vi "AutoRun.vi"() -> ()   [LabVIEW 2012]
uses:
  resultShow.vi
panel:
  in  "布尔":bool
  out "毫秒计时值":u32
  in  "stepMotor/ECU":string
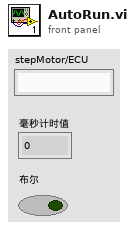
[diagram p1: front panel]
types:
  T1 = cluster{"takesTime":refnum<vi>, "userStatus":refnum<vi>, "userName":refnum<vi>, "connectionMode":refnum<vi>, "productsName":refnum<vi>, "rigStatus":refnum<vi>, "总成扫码":refnum<vi>}
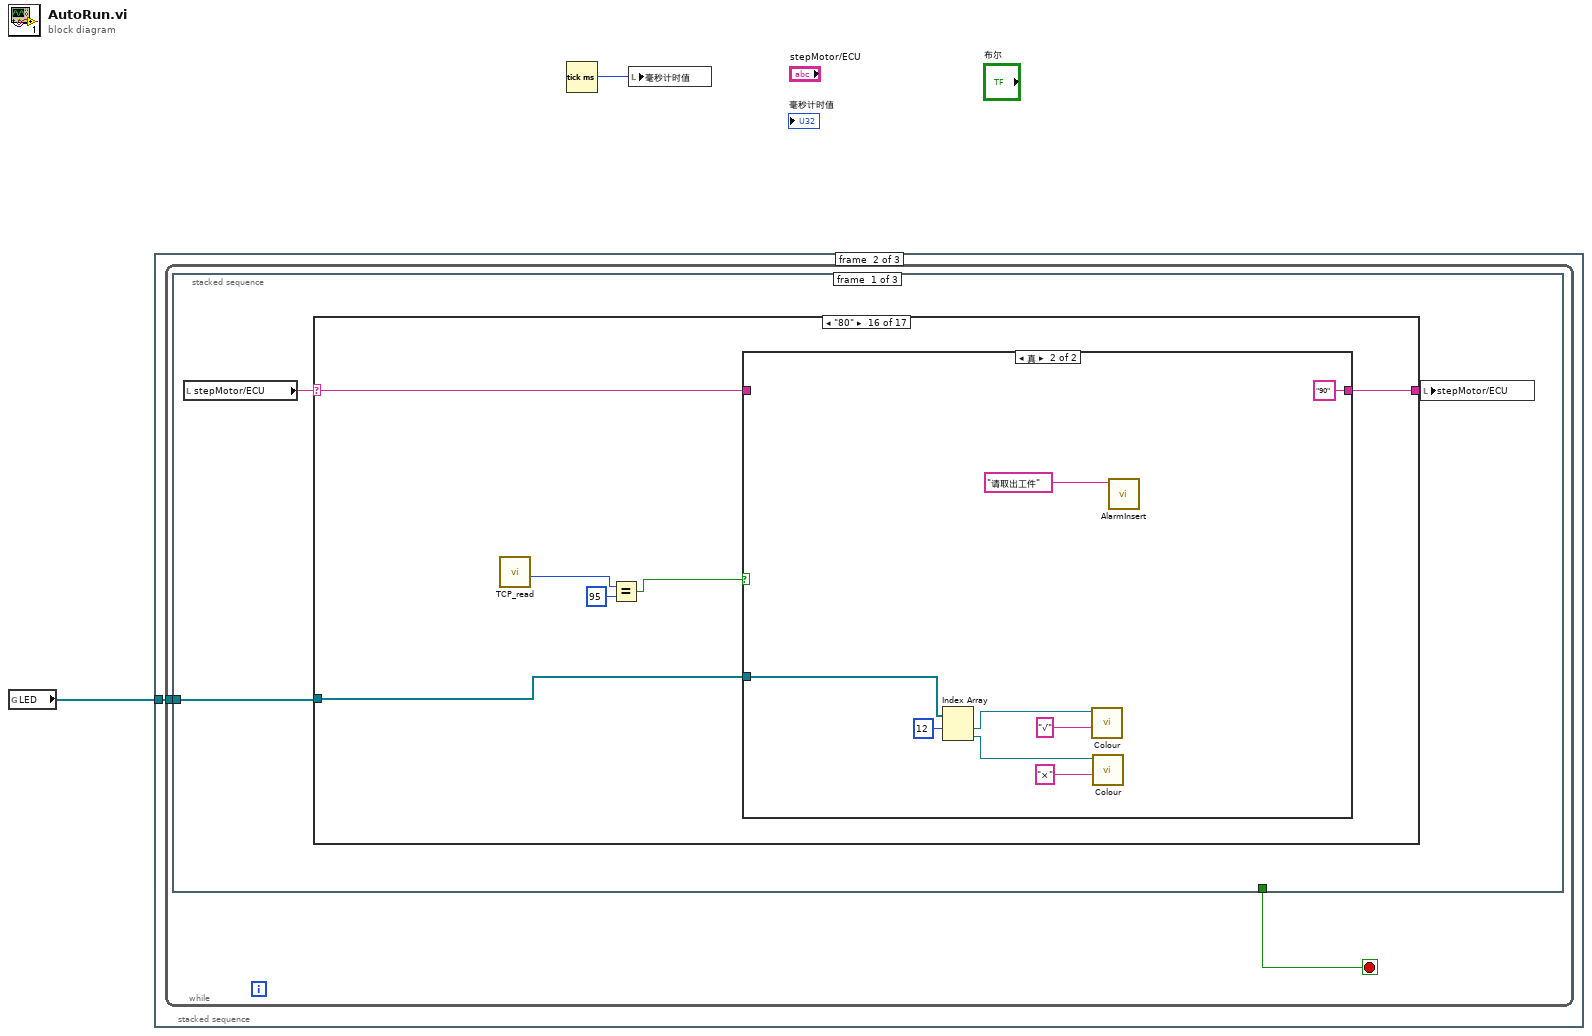
[diagram p0: block diagram]
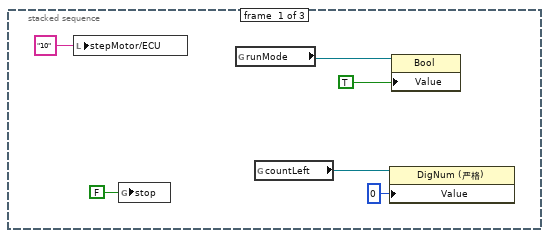
[diagram p2: hidden frame]
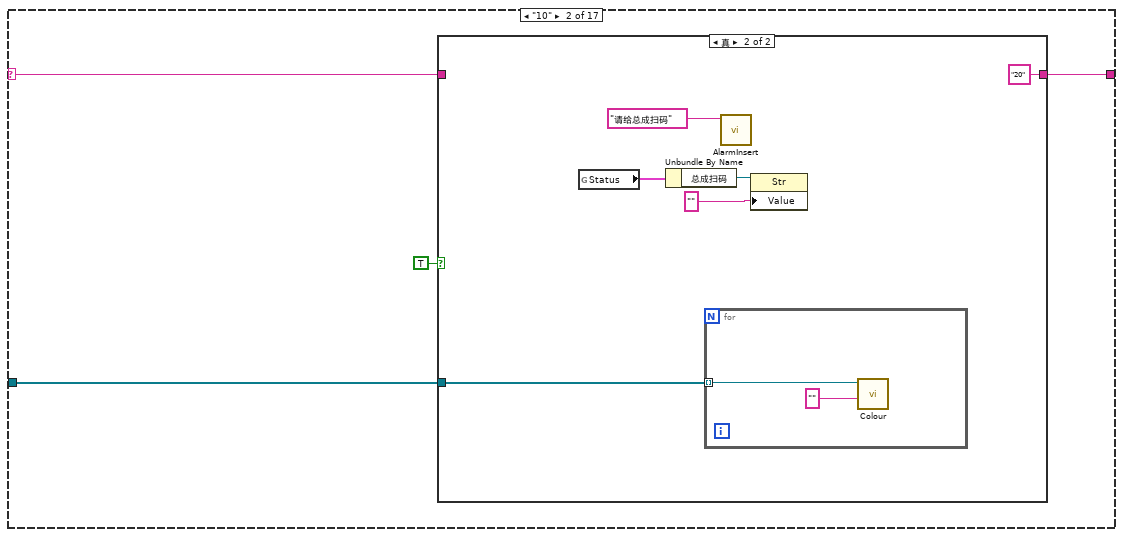
[diagram p4: hidden frame]
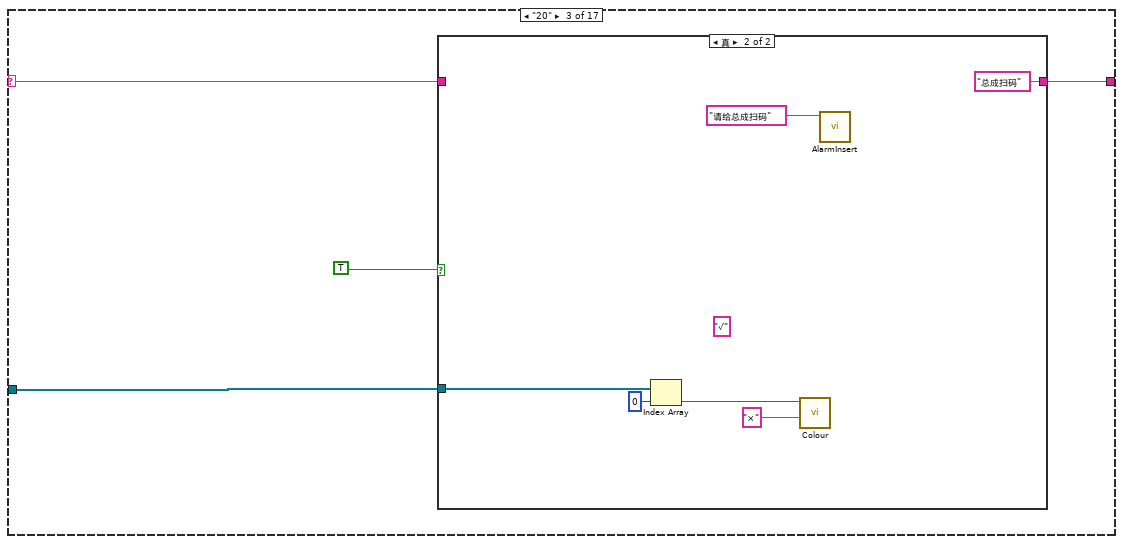
[diagram p6: hidden frame]
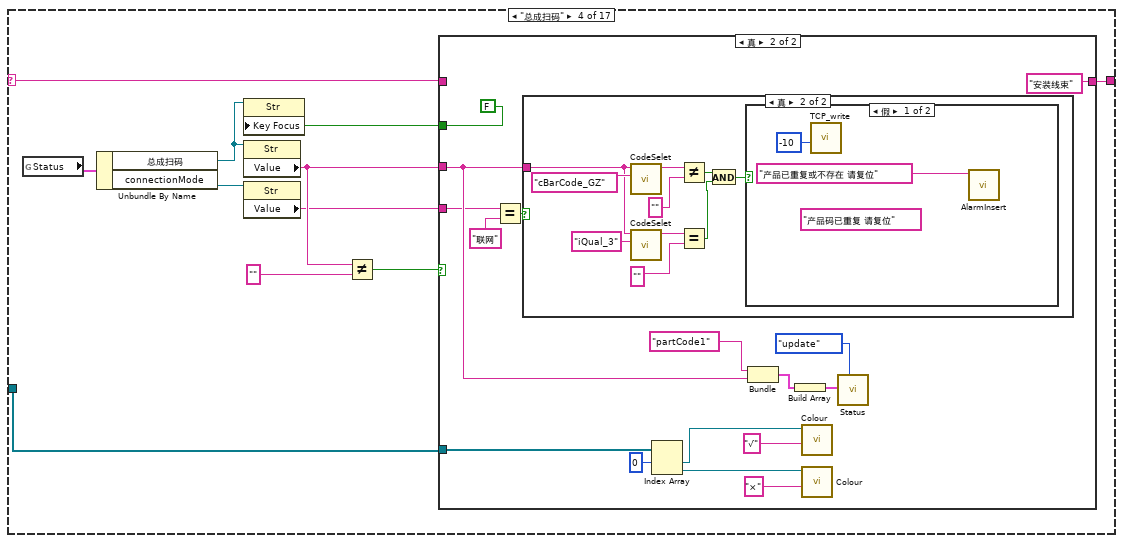
[diagram p8: hidden frame]
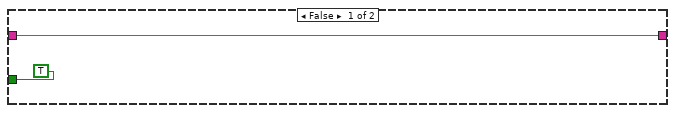
[diagram p9: hidden frame]
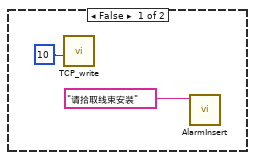
[diagram p10: hidden frame]
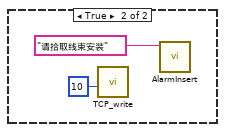
[diagram p11: hidden frame]
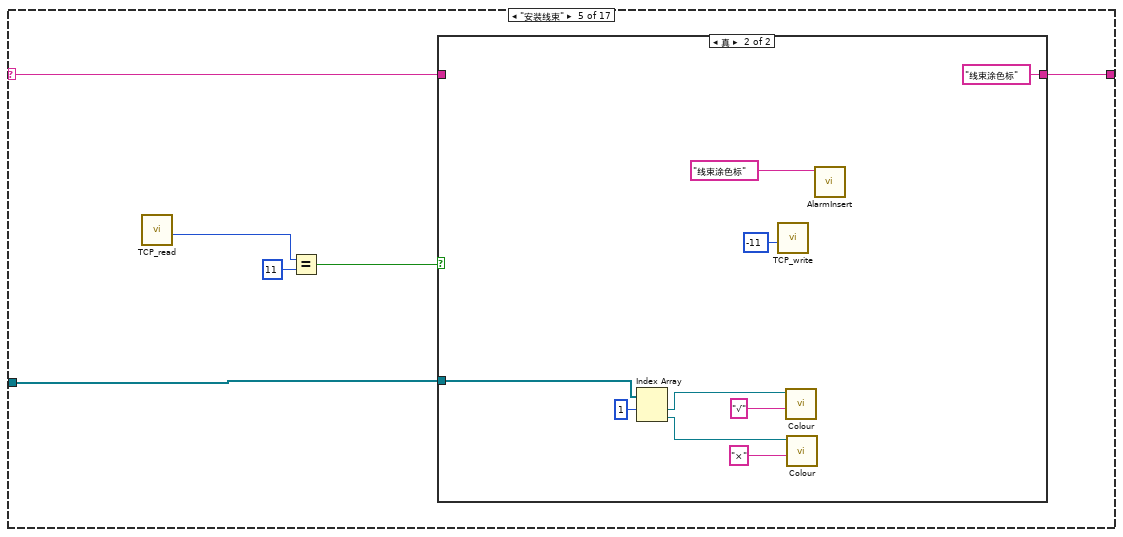
[diagram p12: hidden frame]
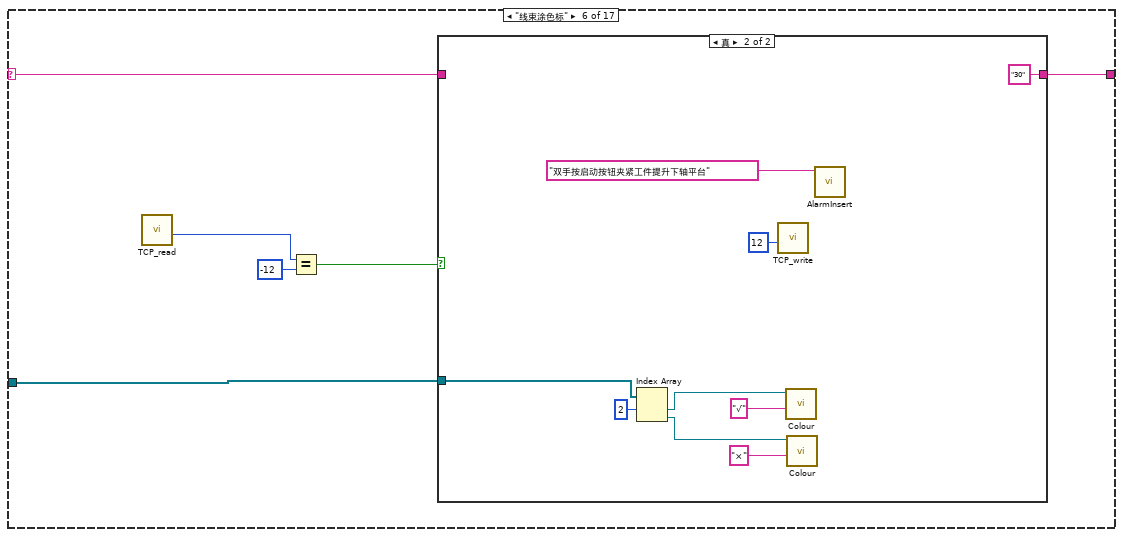
[diagram p14: hidden frame]
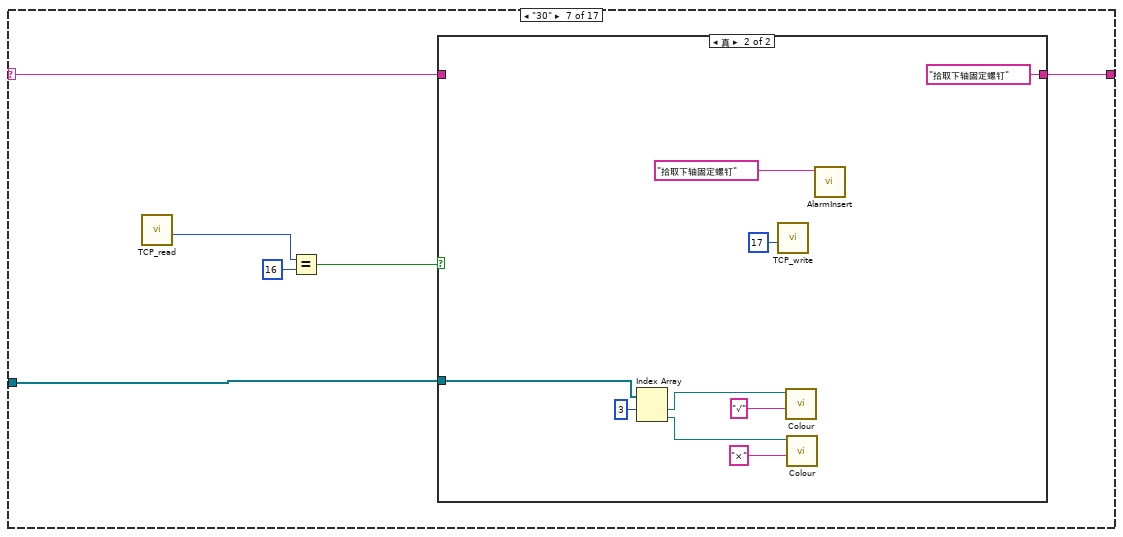
[diagram p16: hidden frame]
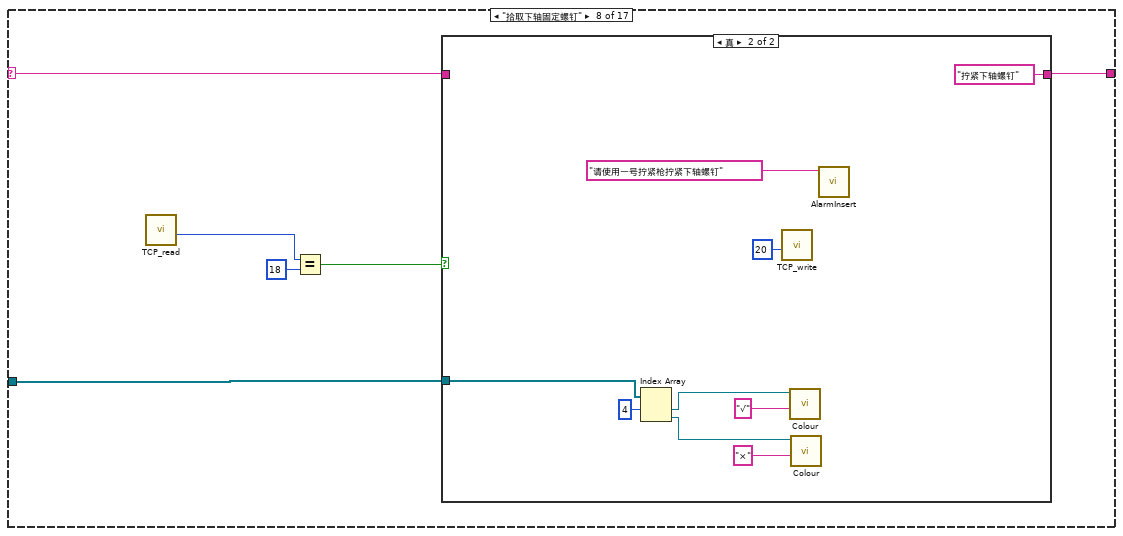
[diagram p18: hidden frame]
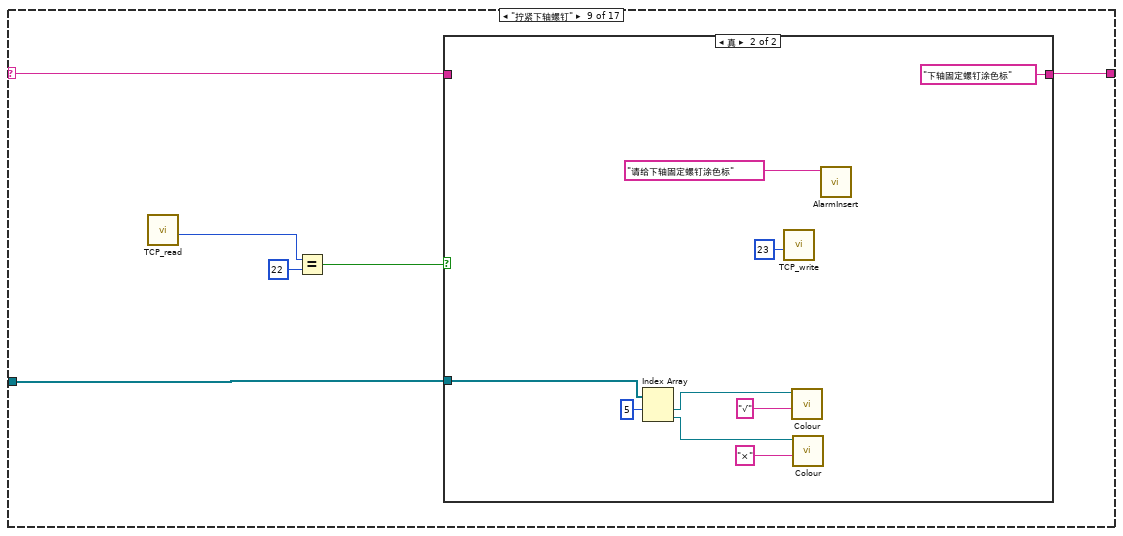
[diagram p20: hidden frame]
diagram:
  n1 = global read "resultShow.vi" "LED"() -> (w2:refnum<vi>[])
  n2 = stacked-sequence {
    tunnel: w2 -> [_ w9 _]
    frame #0 {
      n3 = local write "stepMotor/ECU"("10" ("step")) -> ()
      n4 = global write "全局 3.vi" "stop"(FALSE ("布尔 2")) -> ()
      n5 = global read "resultShow.vi" "runMode"() -> (w5:refnum<vi>)
      n6 = global read "resultShow.vi" "countLeft"() -> (w3:refnum<vi>)
      n7 = property class="DigNum (严格)"(reference=w3, "Value"=u32 0 ("值")) -> ()  [unwired: 1 in, 2 out]
      n8 = property class="Bool"(reference=w5, "Value"=TRUE ("m")) -> ()  [unwired: 1 in, 2 out]
    }
    frame #1 {
      n9 = while {
        tunnel: w9 -> [w10]
        stop <- w11 stop-if-true
        n10 = stacked-sequence {
          tunnel: [_ _ w333] -> w11
          tunnel: w10 -> [w12 _ _]
          frame #0 {
            n11 = local read "stepMotor/ECU"() -> (w13:string)
            n12 = case shown="\"80\"" w13 {
              selector: w13 -> [w15 w18 w31 w46 w89 w105 w121 w134 w150 w167 w185 w201 w217 w231 w247 w274 w289]
              tunnel: [w15 w19 w32 w44 w90 w106 w122 w133 w151 w165 w186 w202 w218 w229 w248 w275 w290] -> w14
              tunnel: w12 -> [_ w16 w30 w45 w85 w101 w117 w135 w149 w166 w181 w197 w213 w230 w246 w270 w285]
              frame "假", Default {
              }
              frame "10" {
                n13 = case shown="真" TRUE {
                  tunnel: [w20 "20"] -> w19
                  tunnel: w18 -> [w20 _]
                  tunnel: w16 -> [_ w25]
                  frame False {
                  }
                  frame True {
                    n14 = global read "resultShow.vi" "Status"() -> (w22:T1)
                    n15 = Unbundle By Name(w22) -> ("总成扫码"=w23:refnum<vi>)
                    n16 = for {
                      tunnel: w25 -> [w27] mode=indexing
                      n17 = call "Colour.vi"("result"="" ("元素"), "colourRef"=w27) -> ()  [unwired: 9 in, 1 out]
                    }
                    n18 = call "AlarmInsert.vi"("消息名"="请给总成扫码") -> ()  [unwired: 11 in]
                    n19 = property class="Str"(reference=w23, "Value"="") -> ()  [unwired: 1 in, 2 out]
                  }
                }
              }
              frame "20" {
                n20 = case shown="真" TRUE {
                  tunnel: [w33 "总成扫码"] -> w32
                  tunnel: w31 -> [w33 _]
                  tunnel: w30 -> [_ w35]
                  frame False {
                  }
                  frame True {
                    (unwired) "√" ("元素")
                    n21 = Index Array(array=w35, index=0 ("索引")) -> (element=w37:refnum<vi>)
                    n22 = call "Colour.vi"("result"="×" ("元素"), "colourRef"=w37) -> ()  [unwired: 9 in, 1 out]
                    n23 = call "AlarmInsert.vi"("消息名"="请给总成扫码") -> ()  [unwired: 11 in]
                  }
                }
              }
              frame "总成扫码" {
                n24 = global read "resultShow.vi" "Status"() -> (w47:T1)
                n25 = Unbundle By Name(w47) -> ("总成扫码"=w49:refnum<vi>, "connectionMode"=w41:refnum<vi>)
                n26 = property class="Str"(reference=w49) -> ("Value"=w43:string)  [unwired: 1 in, 2 out]
                n27 = property class="Str"(reference=w41) -> ("Value"=w40:string)  [unwired: 1 in, 2 out]
                n28 = Not Equal?(x=w43, y="") -> (x != y?=w50:bool)
                n29 = case shown="真" w50 {
                  tunnel: [w52 "安装线束"] -> w44
                  tunnel: w46 -> [w52 _]
                  tunnel: w45 -> [_ w65]
                  tunnel: w43 -> [_ w59]
                  tunnel: [TRUE FALSE] -> w42
                  tunnel: w40 -> [_ w53]
                  frame False {
                  }
                  frame True {
                    n30 = Equal?(x=w53, y="联网") -> (x = y?=w55:bool)
                    n31 = case shown="真" w55 {
                      tunnel: w59 -> [_ w76]
                      frame False {
                        n32 = call "TCP_write.vi"("写入数据"=i8 10) -> ()  [unwired: 11 in]
                        n33 = call "AlarmInsert.vi"("消息名"="请拾取线束安装") -> ()  [unwired: 11 in]
                      }
                      frame True {
                        n34 = call "CodeSelet.vi"("字符串"="cBarCode_GZ" ("code"), "parameter name"=w76) -> ("readData"=w79:string)  [unwired: 9 in]
                        n35 = call "CodeSelet.vi"("字符串"="iQual_3" ("code"), "parameter name"=w76) -> ("readData"=w77:string)  [unwired: 9 in]
                        n36 = Not Equal?(x=w79, y="" ("元素")) -> (x != y?=w74:bool)
                        n37 = Equal?(x=w77, y="" ("元素")) -> (x = y?=w72:bool)
                        n38 = And(x=w74, y=w72) -> (x .and. y?=w73:bool)
                        n39 = case shown="假" w73 {
                          frame False {
                            (unwired) "产品码已重复 请复位" ("string_5")
                            n40 = call "TCP_write.vi"("写入数据"=i8 -10) -> ()  [unwired: 11 in]
                            n41 = call "AlarmInsert.vi"("消息名"="产品已重复或不存在 请复位" ("string_5")) -> ()  [unwired: 11 in]
                          }
                          frame True {
                            n42 = call "TCP_write.vi"("写入数据"=i8 10) -> ()  [unwired: 11 in]
                            n43 = call "AlarmInsert.vi"("消息名"="请拾取线束安装") -> ()  [unwired: 11 in]
                          }
                        }
                      }
                    }
                    n44 = Index Array(array=w65, index #1=0 ("索引")) -> (element #1=w63:refnum<vi>, element #2=w62:refnum<vi>)  [unwired: 1 in]
                    n45 = Bundle("元素"="partCode1", "Value"=w59) -> (w61:cluster{"元素":string, "Value":string})  [unwired: 1 in]
                    n46 = Build Array(w61) -> (w58:cluster{"元素":string, "Value":string}[])
                    n47 = call "Colour.vi"("result"="√" ("元素"), "colourRef"=w63) -> ()  [unwired: 9 in, 1 out]
                    n48 = call "Colour.vi"("result"="×" ("元素"), "colourRef"=w62) -> ()  [unwired: 9 in, 1 out]
                    n49 = call "Status.vi"("模式"=enum16{"select", "insert", "update", "delete"}."update", "nameData"=w58) -> ()  [unwired: 9 in, 1 out]
                  }
                }
                n50 = property class="Str"(reference=w49, "Key Focus"=w42) -> ()  [unwired: 1 in, 2 out]
              }
              frame "安装线束" {
                n51 = call "TCP_read.vi"() -> ("元素"=w88:i8)  [unwired: 10 in, 1 out]
                n52 = Equal?(x=w88, y=i8 11) -> (x = y?=w86:bool)
                n53 = case shown="真" w86 {
                  tunnel: [w91 "线束涂色标"] -> w90
                  tunnel: w89 -> [w91 _]
                  tunnel: w85 -> [_ w92]
                  frame False {
                  }
                  frame True {
                    n54 = Index Array(array=w92, index #1=1 ("索引")) -> (element #1=w96:refnum<vi>, element #2=w93:refnum<vi>)  [unwired: 1 in]
                    n55 = call "TCP_write.vi"("写入数据"=i8 -11) -> ()  [unwired: 11 in]
                    n56 = call "Colour.vi"("result"="√" ("元素"), "colourRef"=w96) -> ()  [unwired: 9 in, 1 out]
                    n57 = call "Colour.vi"("result"="×" ("元素"), "colourRef"=w93) -> ()  [unwired: 9 in, 1 out]
                    n58 = call "AlarmInsert.vi"("消息名"="线束涂色标" ("string_5")) -> ()  [unwired: 11 in]
                  }
                }
              }
              frame "线束涂色标" {
                n59 = call "TCP_read.vi"() -> ("元素"=w104:i8)  [unwired: 10 in, 1 out]
                n60 = Equal?(x=w104, y=i8 -12) -> (x = y?=w102:bool)
                n61 = case shown="真" w102 {
                  tunnel: [w107 "30"] -> w106
                  tunnel: w105 -> [w107 _]
                  tunnel: w101 -> [_ w108]
                  frame False {
                  }
                  frame True {
                    n62 = Index Array(array=w108, index #1=2 ("索引")) -> (element #1=w112:refnum<vi>, element #2=w109:refnum<vi>)  [unwired: 1 in]
                    n63 = call "TCP_write.vi"("写入数据"=i8 12) -> ()  [unwired: 11 in]
                    n64 = call "Colour.vi"("result"="√" ("元素"), "colourRef"=w112) -> ()  [unwired: 9 in, 1 out]
                    n65 = call "Colour.vi"("result"="×" ("元素"), "colourRef"=w109) -> ()  [unwired: 9 in, 1 out]
                    n66 = call "AlarmInsert.vi"("消息名"="双手按启动按钮夹紧工件提升下轴平台" ("string_5")) -> ()  [unwired: 11 in]
                  }
                }
              }
              frame "30" {
                n67 = call "TCP_read.vi"() -> ("元素"=w120:i8)  [unwired: 10 in, 1 out]
                n68 = Equal?(x=w120, y=i8 16) -> (x = y?=w118:bool)
                n69 = case shown="真" w118 {
                  tunnel: [w123 "拾取下轴固定螺钉"] -> w122
                  tunnel: w121 -> [w123 _]
                  tunnel: w117 -> [_ w124]
                  frame False {
                  }
                  frame True {
                    n70 = Index Array(array=w124, index #1=3 ("索引")) -> (element #1=w128:refnum<vi>, element #2=w125:refnum<vi>)  [unwired: 1 in]
                    n71 = call "TCP_write.vi"("写入数据"=i8 17) -> ()  [unwired: 11 in]
                    n72 = call "Colour.vi"("result"="√" ("元素"), "colourRef"=w128) -> ()  [unwired: 9 in, 1 out]
                    n73 = call "Colour.vi"("result"="×" ("元素"), "colourRef"=w125) -> ()  [unwired: 9 in, 1 out]
                    n74 = call "AlarmInsert.vi"("消息名"="拾取下轴固定螺钉" ("string_5")) -> ()  [unwired: 11 in]
                  }
                }
              }
              frame "拾取下轴固定螺钉" {
                n75 = call "TCP_read.vi"() -> ("元素"=w136:i8)  [unwired: 10 in, 1 out]
                n76 = Equal?(x=w136, y=i8 18) -> (x = y?=w138:bool)
                n77 = case shown="真" w138 {
                  tunnel: [w139 "拧紧下轴螺钉"] -> w133
                  tunnel: w134 -> [w139 _]
                  tunnel: w135 -> [_ w140]
                  frame False {
                  }
                  frame True {
                    n78 = Index Array(array=w140, index #1=4 ("索引")) -> (element #1=w144:refnum<vi>, element #2=w141:refnum<vi>)  [unwired: 1 in]
                    n79 = call "TCP_write.vi"("写入数据"=i8 20) -> ()  [unwired: 11 in]
                    n80 = call "Colour.vi"("result"="√" ("元素"), "colourRef"=w144) -> ()  [unwired: 9 in, 1 out]
                    n81 = call "Colour.vi"("result"="×" ("元素"), "colourRef"=w141) -> ()  [unwired: 9 in, 1 out]
                    n82 = call "AlarmInsert.vi"("消息名"="请使用一号拧紧枪拧紧下轴螺钉" ("string_5")) -> ()  [unwired: 11 in]
                  }
                }
              }
              frame "拧紧下轴螺钉" {
                n83 = call "TCP_read.vi"() -> ("元素"=w152:i8)  [unwired: 10 in, 1 out]
                n84 = Equal?(x=w152, y=i8 22) -> (x = y?=w154:bool)
                n85 = case shown="真" w154 {
                  tunnel: [w155 "下轴固定螺钉涂色标"] -> w151
                  tunnel: w150 -> [w155 _]
                  tunnel: w149 -> [_ w156]
                  frame False {
                  }
                  frame True {
                    n86 = Index Array(array=w156, index #1=5 ("索引")) -> (element #1=w160:refnum<vi>, element #2=w157:refnum<vi>)  [unwired: 1 in]
                    n87 = call "TCP_write.vi"("写入数据"=i8 23) -> ()  [unwired: 11 in]
                    n88 = call "Colour.vi"("result"="√" ("元素"), "colourRef"=w160) -> ()  [unwired: 9 in, 1 out]
                    n89 = call "Colour.vi"("result"="×" ("元素"), "colourRef"=w157) -> ()  [unwired: 9 in, 1 out]
                    n90 = call "AlarmInsert.vi"("消息名"="请给下轴固定螺钉涂色标" ("string_5")) -> ()  [unwired: 11 in]
                  }
                }
              }
              frame "下轴固定螺钉涂色标" {
                n91 = call "TCP_read.vi"() -> ("元素"=w168:i8)  [unwired: 10 in, 1 out]
                n92 = Equal?(x=w168, y=i8 24) -> (x = y?=w170:bool)
                n93 = case shown="真" w170 {
                  tunnel: [w171 "40"] -> w165
                  tunnel: w167 -> [w171 _]
                  tunnel: w166 -> [_ w172]
                  frame False {
                  }
                  frame True {
                    n94 = Index Array(array=w172, index #1=6 ("索引")) -> (element #1=w176:refnum<vi>, element #2=w173:refnum<vi>)  [unwired: 1 in]
                    n95 = call "TCP_write.vi"("写入数据"=i8 25) -> ()  [unwired: 11 in]
                    n96 = call "Colour.vi"("result"="√" ("元素"), "colourRef"=w176) -> ()  [unwired: 9 in, 1 out]
                    n97 = call "Colour.vi"("result"="×" ("元素"), "colourRef"=w173) -> ()  [unwired: 9 in, 1 out]
                    n98 = call "AlarmInsert.vi"("消息名"="请将下轴翻起后按左启动键复位下轴平台" ("string_5")) -> ()  [unwired: 11 in]
                  }
                }
              }
              frame "40" {
                n99 = call "TCP_read.vi"() -> ("元素"=w184:i8)  [unwired: 10 in, 1 out]
                n100 = Equal?(x=w184, y=i8 31) -> (x = y?=w182:bool)
                n101 = case shown="真" w182 {
                  tunnel: [w187 "50"] -> w186
                  tunnel: w185 -> [w187 _]
                  tunnel: w181 -> [_ w188]
                  frame False {
                  }
                  frame True {
                    n102 = Index Array(array=w188, index #1=7 ("索引")) -> (element #1=w192:refnum<vi>, element #2=w189:refnum<vi>)  [unwired: 1 in]
                    n103 = call "TCP_write.vi"("写入数据"=i8 40) -> ()  [unwired: 11 in]
                    n104 = call "AlarmInsert.vi"("消息名"="双手按启动按钮启动翻转" ("string_5")) -> ()  [unwired: 11 in]
                    n105 = call "Colour.vi"("result"="√" ("元素"), "colourRef"=w192) -> ()  [unwired: 9 in, 1 out]
                    n106 = call "Colour.vi"("result"="×" ("元素"), "colourRef"=w189) -> ()  [unwired: 9 in, 1 out]
                  }
                }
              }
              frame "50" {
                n107 = call "TCP_read.vi"() -> ("元素"=w200:i8)  [unwired: 10 in, 1 out]
                n108 = Equal?(x=w200, y=i8 43) -> (x = y?=w198:bool)
                n109 = case shown="真" w198 {
                  tunnel: [w203 "60"] -> w202
                  tunnel: w201 -> [w203 _]
                  tunnel: w197 -> [_ w204]
                  frame False {
                  }
                  frame True {
                    n110 = Index Array(array=w204, index #1=8 ("索引")) -> (element #1=w208:refnum<vi>, element #2=w205:refnum<vi>)  [unwired: 1 in]
                    n111 = call "TCP_write.vi"("写入数据"=i8 50) -> ()  [unwired: 11 in]
                    n112 = call "Colour.vi"("result"="√" ("元素"), "colourRef"=w208) -> ()  [unwired: 9 in, 1 out]
                    n113 = call "Colour.vi"("result"="×" ("元素"), "colourRef"=w205) -> ()  [unwired: 9 in, 1 out]
                    n114 = call "AlarmInsert.vi"("消息名"="请向左边转两圈以上" ("string_5")) -> ()  [unwired: 11 in]
                  }
                }
              }
              frame "60" {
                n115 = call "TCP_read.vi"() -> ("元素"=w216:i8)  [unwired: 10 in, 1 out]
                n116 = Equal?(x=w216, y=i8 51) -> (x = y?=w214:bool)
                n117 = case shown="真" w214 {
                  tunnel: [w219 "61"] -> w218
                  tunnel: w217 -> [w219 _]
                  tunnel: w213 -> [_ w220]
                  frame False {
                  }
                  frame True {
                    n118 = Index Array(array=w220, index #1=9 ("索引")) -> (element #1=w224:refnum<vi>, element #2=w221:refnum<vi>)  [unwired: 1 in]
                    n119 = call "TCP_write.vi"("写入数据"=i8 60) -> ()  [unwired: 11 in]
                    n120 = call "Colour.vi"("result"="√" ("元素"), "colourRef"=w224) -> ()  [unwired: 9 in, 1 out]
                    n121 = call "Colour.vi"("result"="×" ("元素"), "colourRef"=w221) -> ()  [unwired: 9 in, 1 out]
                    n122 = call "AlarmInsert.vi"("消息名"="请向右边转两圈以上" ("string_5")) -> ()  [unwired: 11 in]
                  }
                }
              }
              frame "61" {
                n123 = call "TCP_read.vi"() -> ("元素"=w234:i8)  [unwired: 10 in, 1 out]
                n124 = Equal?(x=w234, y=i8 61) -> (x = y?=w232:bool)
                n125 = case shown="真" w232 {
                  tunnel: [w235 "70"] -> w229
                  tunnel: w231 -> [w235 _]
                  tunnel: w230 -> [_ w236]
                  frame False {
                  }
                  frame True {
                    n126 = Index Array(array=w236, index #1=10 ("索引")) -> (element #1=w240:refnum<vi>, element #2=w237:refnum<vi>)  [unwired: 1 in]
                    n127 = call "TCP_write.vi"("写入数据"=i8 62) -> ()  [unwired: 11 in]
                    n128 = call "Colour.vi"("result"="√" ("元素"), "colourRef"=w240) -> ()  [unwired: 9 in, 1 out]
                    n129 = call "Colour.vi"("result"="×" ("元素"), "colourRef"=w237) -> ()  [unwired: 9 in, 1 out]
                    n130 = call "AlarmInsert.vi"("消息名"="请判断是否合格" ("string_5")) -> ()  [unwired: 11 in]
                  }
                }
              }
              frame "70" {
                n131 = call "TCP_read.vi"() -> ("元素"=w245:i8)  [unwired: 10 in, 1 out]
                n132 = case shown="72" w245 {
                  tunnel: [w249 w252 w261 "80"] -> w248
                  tunnel: w247 -> [w249 w252 w261 _]
                  tunnel: w246 -> [_ w253 w262 _]
                  frame Default {
                  }
                  frame 71 {
                    n133 = Index Array(array=w253, index #1=11 ("索引")) -> (element #1=w257:refnum<vi>, element #2=w254:refnum<vi>)  [unwired: 1 in]
                    n134 = global write "全局 3.vi" "总合格状态"("" ("元素")) -> ()
                    n135 = global write "全局 3.vi" "合格判断"("√" ("元素")) -> ()
                    n136 = call "Colour.vi"("result"="√" ("元素"), "colourRef"=w257) -> ()  [unwired: 9 in, 1 out]
                    n137 = call "Colour.vi"("result"="×" ("元素"), "colourRef"=w254) -> ()  [unwired: 9 in, 1 out]
                    n138 = call "AlarmInsert.vi"("消息名"="合格 请拆卸下轴后双手按启动按钮" ("string_5")) -> ()  [unwired: 11 in]
                  }
                  frame 72 {
                    w260 = "×" ("元素")
                    n139 = Index Array(array=w262, index #1=11 ("索引")) -> (element #1=w266:refnum<vi>, element #2=w263:refnum<vi>)  [unwired: 1 in]
                    n140 = global write "全局 3.vi" "总合格状态"(w260) -> ()
                    n141 = global write "全局 3.vi" "合格判断"(w260) -> ()
                    n142 = call "Colour.vi"("result"="×" ("元素"), "colourRef"=w266) -> ()  [unwired: 9 in, 1 out]
                    n143 = call "Colour.vi"("result"="×" ("元素"), "colourRef"=w263) -> ()  [unwired: 9 in, 1 out]
                    n144 = call "AlarmInsert.vi"("消息名"="不合格 请拆卸下轴后双手按启动按钮" ("string_5")) -> ()  [unwired: 11 in]
                  }
                  frame 81 {
                  }
                }
              }
              frame "80" {
                n145 = call "TCP_read.vi"() -> ("元素"=w273:i8)  [unwired: 10 in, 1 out]
                n146 = Equal?(x=w273, y=i8 95) -> (x = y?=w271:bool)
                n147 = case shown="真" w271 {
                  tunnel: [w276 "90"] -> w275
                  tunnel: w274 -> [w276 _]
                  tunnel: w270 -> [_ w278]
                  frame False {
                  }
                  frame True {
                    n148 = Index Array(array=w278, index #1=12 ("索引")) -> (element #1=w282:refnum<vi>, element #2=w279:refnum<vi>)  [unwired: 1 in]
                    n149 = call "Colour.vi"("result"="√" ("元素"), "colourRef"=w282) -> ()  [unwired: 9 in, 1 out]
                    n150 = call "Colour.vi"("result"="×" ("元素"), "colourRef"=w279) -> ()  [unwired: 9 in, 1 out]
                    n151 = call "AlarmInsert.vi"("消息名"="请取出工件" ("string_5")) -> ()  [unwired: 11 in]
                  }
                }
              }
              frame "90" {
                n152 = call "TCP_read.vi"() -> ("元素"=w288:i8)  [unwired: 10 in, 1 out]
                n153 = Equal?(x=w288, y=i8 95) -> (x = y?=w286:bool)
                n154 = case shown="真" w286 {
                  tunnel: [w291 "10"] -> w290
                  tunnel: w289 -> [w291 _]
                  tunnel: w285 -> [_ w310]
                  frame False {
                  }
                  frame True {
                    n155 = global read "resultShow.vi" "Status"() -> (w303:T1)
                    n156 = global read "resultShow.vi" "countLeft"() -> (w309:refnum<vi>)
                    n157 = local read "毫秒计时值"() -> (w294:u32)
                    n158 = Tick Count (ms)() -> (millisecond timer value=w292:u32)
                    n159 = Unbundle By Name(w303) -> ("connectionMode"=w304:refnum<vi>)
                    n160 = Index Array(array=w310, index=13 ("索引")) -> (element=w312:refnum<vi>)
                    n161 = Subtract(x=w292, y=w294) -> (x-y=w298:u32)
                    n162 = property class="DigNum (严格)"(reference=w309) -> (reference out=w308:refnum<vi>, "Value"=w307:u32)  [unwired: 1 in, 1 out]
                    n163 = Divide(x=w298, y=u32 1000) -> (x/y=w296:dbl)
                    n164 = property class="Str"(reference=w304) -> ("Value"=w301:string)  [unwired: 1 in, 2 out]
                    n165 = To Time Stamp(1:w296) -> (0:w295:timestamp)
                    n166 = call "Colour.vi"("result"="√" ("元素"), "colourRef"=w312) -> ()  [unwired: 9 in, 1 out]
                    n167 = Format Date/Time String(seconds (now)=w295) -> (date/time string=w293:string)  [unwired: 2 in]
                    n168 = Increment(x=w307) -> (x+1=w306:u32)
                    n169 = Equal?(x=w301, y="联网") -> (x = y?=w302:bool)
                    n170 = case shown="真" w302 {
                      frame False {
                      }
                      frame True {
                        n171 = call "updateiqual.vi"() -> ()  [unwired: 11 in]
                      }
                    }
                    n172 = property class="DigNum (严格)"(reference=w308, "Value"=w306) -> ()  [unwired: 1 in, 2 out]
                    n173 = call "AlarmInsert.vi"("takesTime"=w293, "消息名"="完成取回工件！" ("string_5")) -> ()  [unwired: 10 in]
                    n174 = call "TCP_write.vi"("写入数据"=i8 96) -> ()  [unwired: 11 in]
                  }
                }
              }
            }
            n175 = local write "stepMotor/ECU"(w14) -> ()
          }
          frame #1 {
            n176 = call "TCP_read.vi"() -> ("元素"=w318:i8)  [unwired: 10 in, 1 out]
            n177 = local read "布尔"() -> (w315:bool)
            n178 = local read "stepMotor/ECU"() -> (w320:string)
            n179 = Equal?(x=w318, y=i8 -100) -> (x = y?=w317:bool)
            n180 = Or(x=w317, y=w315) -> (x .or. y?=w316:bool)
            n181 = case shown="真" w316 {
              tunnel: [w322 w329] -> w319
              tunnel: w320 -> [w322 w324]
              frame False {
              }
              frame True {
                n182 = call "TCP_read.vi"() -> ("元素"=w326:i8)  [unwired: 10 in, 1 out]
                n183 = local write "布尔"(TRUE ("布尔")) -> ()
                n184 = Equal?(x=w326, y=i8 0) -> (x = y?=w325:bool)
                n185 = call "AlarmInsert.vi"("消息名"="复位中" ("string_5")) -> ()  [unwired: 11 in]
                n186 = case shown="真" w325 {
                  tunnel: [w330 "10"] -> w329
                  tunnel: w324 -> [w330 _]
                  frame False {
                  }
                  frame True {
                    n187 = local write "布尔"(FALSE ("布尔")) -> ()
                  }
                }
              }
            }
            n188 = local write "stepMotor/ECU"(w319) -> ()
          }
          frame #2 {
            n189 = global read "全局 3.vi" "stop"() -> (w333:bool)
            n190 = Wait (ms)(milliseconds to wait=u32 10 ("等待时间（毫秒）")) -> ()  [unwired: 1 out]
          }
        }
      }
    }
    frame #2 {
      n191 = global read "resultShow.vi" "runMode"() -> (w336:refnum<vi>)
      n192 = property class="Bool"(reference=w336, "Value"=FALSE ("m")) -> ()  [unwired: 1 in, 2 out]
    }
  }
  n193 = Tick Count (ms)() -> (millisecond timer value=w1:u32)
  n194 = local write "毫秒计时值"(w1) -> ()
